vi "ctx avg retry count for device.vi"(10 "device_id":u32, 11 "context":u32) -> (2 "function return":i32, 3 "context out":u32)   [LabVIEW 2019, in "apdm.lvlib"]
doc: "APDM_EXPORT int apdm_ctx_avg_retry_count_for_device(apdm_ctx_t context, const uint32_t device_id);"
uses:
  apdm.lvlib
  Lee Lab/CP FES Walking 2018/Code/Working/LabVIEW/apdm.dll
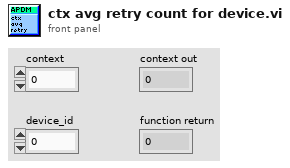
[diagram p1: front panel]
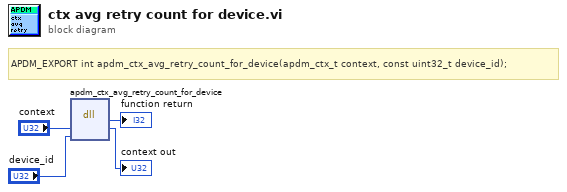
[diagram p0: block diagram]
diagram:
  # "APDM_EXPORT int apdm_ctx_avg_retry_count_for_device(apdm_ctx_t context, const uint32_t device_id);"
  n1 = dll-call lib="C:/Users/jfalesi/Dropbox/Lee Lab/CP FES Walking 2018/Code/Working/LabVIEW/apdm.*" fn="apdm_ctx_avg_retry_count_for_device"("context"="context", "device_id"="device_id") -> (→"function return":i32, "context"=→"context out":u32)  [unwired: 4 in, 2 out]
